vi "Set Boolean Type.vi"(6 "Mouse Position":T1, 7 "User VI Ref":refnum<vi>, 8 "Is Multi-select?":bool, 9 "Remaining Items":refnum<vi>[](array[refnum]), 10 "Affected Items":T8, 11 "Menu Refnum":refnum<k9>) -> (3 "Menu Items To Add":T2[](array[typedef]))   [LabVIEW 2021]
doc: "This implementation of the right click menu VI will set the \"Boolean Type\" for a given Boolean control(s) for a VI. It will categorize the type of the button that is being used so that Theme-ing can be applied appropriately.\n\n<b>Original</b>: This VI is part of a plug-in for modifying the LabVIEW shortcut menus. This is the builder VI which is called when the shortcut menu is built. It tells LabVIEW which shortcut menu items to add to the menu."
uses:
  <resource>/plugins/PopupMenus/support/Shortcut Menu Item Definition.ctl
  <resource>/plugins/PopupMenus/support/Transaction Control.ctl
  <resource>/plugins/PopupMenus/support/Position In Menu.ctl
  <resource>/plugins/PopupMenus/support/Relative Position.ctl
  <resource>/plugins/PopupMenus/support/Checkmark Status.ctl
  <resource>/plugins/PopupMenus/support/Enabled Menu Item Status.ctl
  Set Boolean Type.ctl
  <vilib>/Utility/miscctls.llb/LVPositionTypeDef.ctl
  1857561c-2c4f-473e-aded-e0aee2b8ec2d.vi
panel:
  # "Rules a popup plug-in must follow:\n* This VI's file name must match the file name of the LLB -- only the file extensions should be different.\n* This VI must have debugging disabled or it will be ignored as a plug-in.\n* For all menu items, \"tag suffix + file name of this VI\" must be less than 240 characters.\n* You can disconnect the \"Affected Items\" from the typedef to make the plug-in load faster. The typedef is only there to assist you in keeping this VI and the execution VI using to the same type.\n* All controls on this panel except \"Affected Items\" are locked to prevent accidental edits. Do not change the types or the names of controls other than the elements inside the \"Affected Items\" cluster.\n* See Context Help for more information on the individual controls."
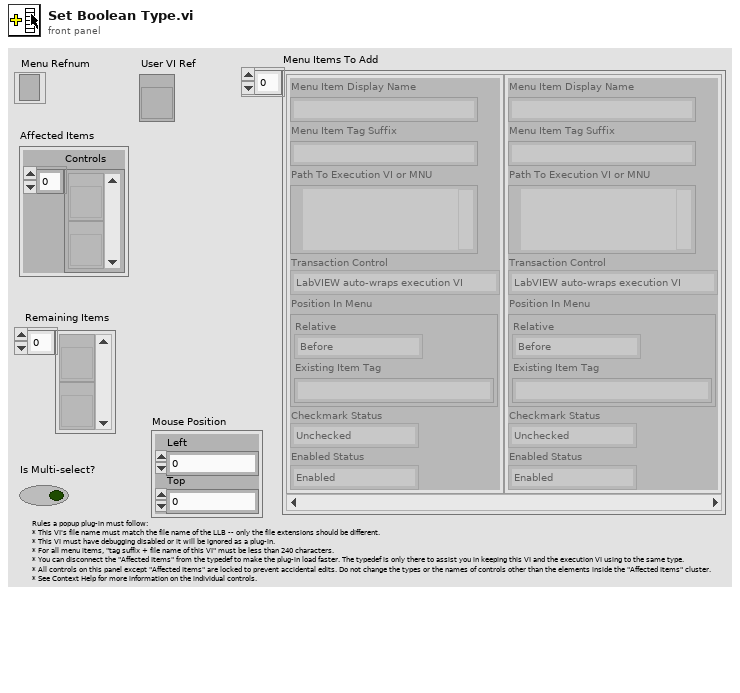
[diagram p1: front panel]
types:
  T1 = typedef "LVPositionTypeDef.ctl" = cluster{"Left":i32, "Top":i32}
  T2 = typedef "Shortcut Menu Item Definition.ctl" = cluster{"Menu Item Display Name":string, "Menu Item Tag Suffix":string, "Path To Execution VI or MNU":path, "Transaction Control":T3, "Position In Menu":T4, "Checkmark Status":T6, "Enabled Status":T7}
  T3 = typedef "Transaction Control.ctl" = enum8{"LabVIEW auto-wraps execution VI", "Execution VI will define if needed"}
  T4 = typedef "Position In Menu.ctl" = cluster{"Relative":T5, "Existing Item Tag":string}
  T5 = typedef "Relative Position.ctl" = enum8{"Before", "Instead of", "After", "Into Submenu"}
  T6 = typedef "Checkmark Status.ctl" = enum8{"Unchecked", "Checked"}
  T7 = typedef "Enabled Menu Item Status.ctl" = enum8{"Enabled", "Disabled"}
  T8 = typedef "Set Boolean Type.ctl" = cluster{"Controls":refnum<vi>[]}
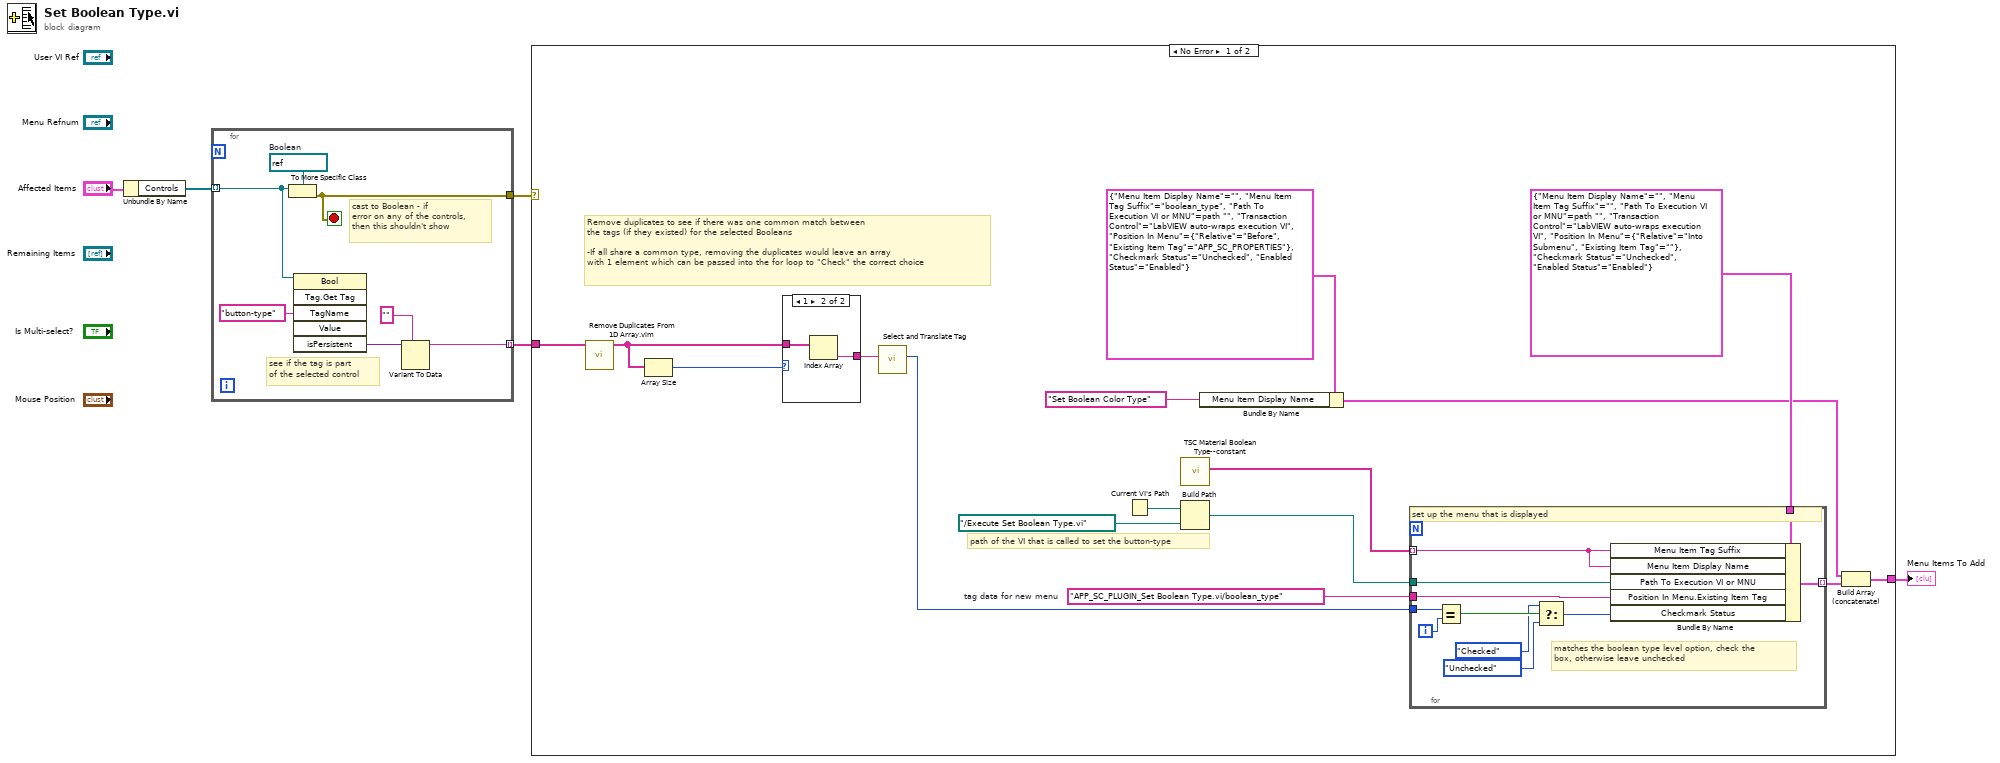
[diagram p0: block diagram]
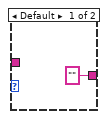
[diagram p2: hidden frame]
diagram:
  n1 = Unbundle By Name("Affected Items") -> ("Controls"=w4:refnum<vi>[])
  n2 = for {
    tunnel: w4 -> [w6] mode=indexing
    tunnel: [w11] -> w3
    tunnel: [w7] -> w1 mode=indexing
    stop <- w11 stop-if-true
    w12 = refnum<vi> refnum  # Boolean
    # "cast to Boolean - if\nerror on any of the controls, \nthen this shouldn't show"
    # "see if the tag is part \nof the selected control"
    n3 = To More Specific Class(target class=w12, reference=w6) -> (error out=w11:errorcluster)  [unwired: 1 in, 1 out]
    n4 = invoke class="Bool" method="Tag.Get Tag"(reference=w6, "TagName"="button-type" ("Tag Name")) -> ("isPersistent"=w9:variant)  [unwired: 4 in, 5 out]
    n5 = Variant To Data(type="", Variant=w9) -> (data=w7:string)  [unwired: 1 in, 1 out]
  }
  n6 = case shown="No Error" w3 {
    tunnel: [w15 _] -> w2
    tunnel: w1 -> [w23 _]
    frame No Error {
      w13 = "APP_SC_PLUGIN_Set Boolean Type.vi/boolean_type"  # tag data for new menu
      # "Remove duplicates to see if there was one common match between\nthe tags (if they existed) for the selected Booleans\n\n-If all share a common type, removing the duplicates would leave an array\nwith 1 element which can be passed into the for loop to \"Check\" the correct choice"
      # "path of the VI that is called to set the button-type"
      n7 = call "Remove Duplicates From 1D Array.vim"("array"=w23) -> ("array with duplicates removed"=w21:string[])  [unwired: 10 in]
      n8 = Array Size(array=w21) -> (size(s)=w22:i32)
      n9 = case shown="1" w22 {
        tunnel: w21 -> [_ w31]
        tunnel: ["" w30] -> w19
        frame Default {
        }
        frame 1 {
          n10 = Index Array(array=w31) -> (element=w30:string)  [unwired: 1 in]
        }
      }
      n11 = call "Select and Translate Tag.vi"("Current Item"=w19) -> ("index of element"=w18:i32)  [unwired: 10 in]
      n12 = Current VI's Path() -> (path=w27:path)
      n13 = call "TSC Material Boolean Type--constant.vi"() -> ("boolean types"=w20:string[])  [unwired: 11 in]
      n14 = Build Path(base path=w27, name or relative path=path "../Execute Set Boolean Type.vi" ("execute path")) -> (appended path=w26:path)
      n15 = Bundle By Name(cluster=T2 {"Menu Item Display Name"="", "Menu Item Tag Suffix"="boolean_type", "Path To Execution VI or MNU"=path "", "Transaction Control"=enum."LabVIEW auto-wraps execution VI", "Position In Menu"={"Relative"=enum."Before", "Existing Item Tag"="APP_SC_PROPERTIES"}, "Checkmark Status"=enum."Unchecked", "Enabled Status"=enum."Enabled"} ("Cluster"), "Menu Item Display Name"="Set Boolean Color Type" ("Boolean Type Level")) -> (w14:T2)
      n16 = for {
        tunnel: T2 {"Menu Item Display Name"="", "Menu Item Tag Suffix"="", "Path To Execution VI or MNU"=path "", "Transaction Control"=enum."LabVIEW auto-wraps execution VI", "Position In Menu"={"Relative"=enum."Into Submenu", "Existing Item Tag"=""}, "Checkmark Status"=enum."Unchecked", "Enabled Status"=enum."Enabled"} ("Cluster") -> [w42]
        tunnel: [w41] -> w24 mode=indexing
        tunnel: w26 -> [w40]
        tunnel: w13 -> [w39]
        tunnel: w20 -> [w34] mode=indexing
        tunnel: w18 -> [w33]
        i -> [w32]
        # "matches the boolean type level option, check the \nbox, otherwise leave unchecked"
        # "set up the menu that is displayed"
        n17 = Equal?(x=w33, y=w32) -> (x = y?=w38:bool)
        n18 = Select(t=Checkmark_Status."Checked" ("Checkmark Status"), s=w38, f=Checkmark_Status."Unchecked" ("Checkmark Status")) -> (s? t:f=w35:T6)
        n19 = Bundle By Name(cluster=w42, "Menu Item Tag Suffix"=w34, "Menu Item Display Name"=w34, "Path To Execution VI or MNU"=w40, "Position In Menu.Existing Item Tag"=w39, "Checkmark Status"=w35) -> (w41:T2)
      }
      n20 = Build Array (concatenate)(w14, w24) -> (w15:T2[])
    }
    frame Error {
    }
  }
  "Menu Items To Add" <- w2
